vi "Compile Initially Connected Endpoints for Module.vi"(6 "Module":string, 8 "error in":errorcluster, 9 "Initially Connected Endpoints":T2[](array[typedef]), 10 "Communication Configuration":T3, 11 "Compiled Connections Buffer":T1[](array[typedef])) -> (0 "error out":errorcluster, 3 "Compiled Initial Connection Indices":i32[](array[numeric]))   [LabVIEW 2020, in "Routing and Faulting System Explorer.lvlib"]
uses:
  Routing and Faulting System Explorer.lvlib
  Shared/Communication Configuration.ctl
  Shared/Routing and Faulting Hardware API/Types/Connection.ctl
  Shared/Compiled Connection.ctl
  Shared/Connection.ctl
  Shared/Routing and Faulting Shared.lvlib
  Shared/Routing and Faulting Hardware API/Routing and Faulting Hardware API.lvlib
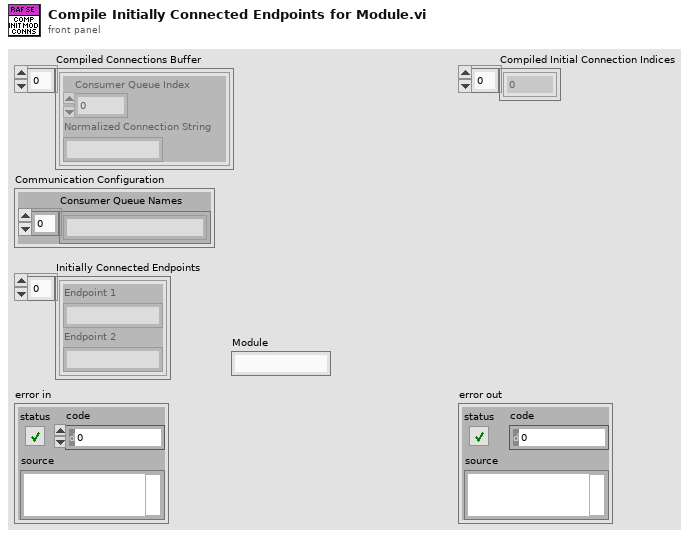
[diagram p1: front panel]
types:
  T1 = typedef "Routing and Faulting Shared.lvlib/Compiled Connection.ctl" = cluster{"Consumer Queue Index":i32, "Normalized Connection String":string}
  T2 = typedef "Routing and Faulting Hardware API.lvlib/Connection.ctl" = cluster{"Endpoint 1":string, "Endpoint 2":string}
  T3 = typedef "Routing and Faulting Shared.lvlib/Communication Configuration.ctl" = cluster{"Consumer Queue Names":string[]}
  T4 = typedef "Routing and Faulting Shared.lvlib/Connection.ctl" = cluster{"Module":string, "Source":string, "Destination":string}
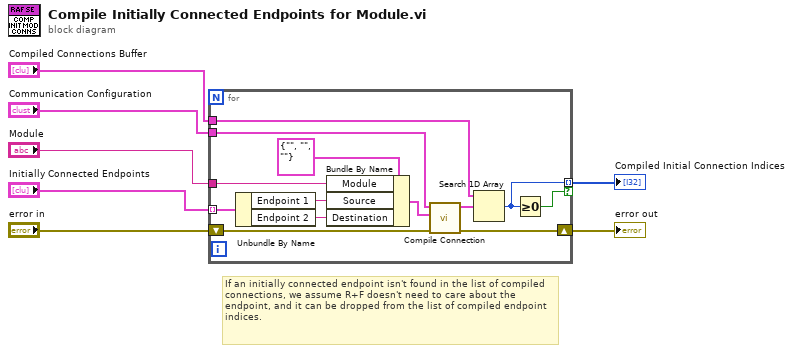
[diagram p0: block diagram]
diagram:
  # "If an initially connected endpoint isn't found in the list of compiled connections, we assume R+F doesn't need to care about the endpoint, and it can be dropped from the list of compiled endpoint indices."
  n1 = for {
    tunnel: "Initially Connected Endpoints" -> [w20] mode=indexing
    tunnel: "Communication Configuration" -> [w15]
    shift-right: [w14] -> w2
    shift-left: "error in" -> [w13]
    tunnel: "Compiled Connections Buffer" -> [w12]
    tunnel: "Module" -> [w10]
    tunnel: [w9] -> w1 mode=indexing if=w8
    n2 = Unbundle By Name(w20) -> ("Endpoint 1"=w17:string, "Endpoint 2"=w16:string)
    n3 = Bundle By Name(cluster=T4 {"Module"="", "Source"="", "Destination"=""} ("Connection"), "Module"=w10, "Source"=w17, "Destination"=w16) -> (w18:T4)
    n4 = call "Compile Connection.vi"("error in (no error)"=w13, "Connection"=w18, "Communication Configuration"=w15) -> ("error out"=w14:errorcluster, "Compiled Connection"=w11:T1)  [unwired: 7 in]
    n5 = Search 1D Array(1D array=w12, element=w11) -> (index of element=w9:i32)  [unwired: 1 in]
    n6 = Greater Or Equal To 0?(x=w9) -> (x >= 0?=w8:bool)
  }
  "error out" <- w2
  "Compiled Initial Connection Indices" <- w1
